vi "Bundle.vi"(8 "error in (no error)":errorcluster, 10 "Actor":refnum<class "Actor.lvclass">, 11 "Launch Subscriber Msg in":refnum<class "Launch Subscriber Msg.lvclass">) -> (0 "error out":errorcluster, 3 "Launch Subscriber Msg out":refnum<class "Launch Subscriber Msg.lvclass">)   [LabVIEW 2020, in "Publisher.lvlib" / "Launch Subscriber Msg.lvclass"]
doc: "Populate the Launc Subscriber Msg class."
uses:
  Launch Subscriber Msg.lvclass
  PPL/HDH.Actor Framework.Core.Actor.lvlibp/1abvi3w/vi.lib/ActorFramework/Actor/Actor.lvclass
  Launch Subscriber Msg.lvclass/Launch Subscriber Msg.ctl
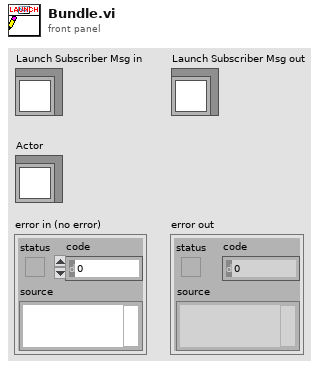
[diagram p1: front panel]
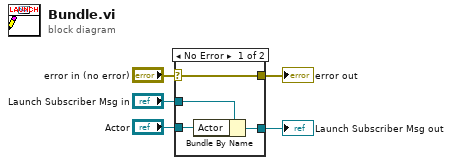
[diagram p0: block diagram]
diagram:
  n1 = case shown="No Error" "error in (no error)" {
    selector: "error in (no error)" -> [w9 w10]
    tunnel: [w9 w10] -> w4
    tunnel: [w7 w11] -> w2
    tunnel: "Launch Subscriber Msg in" -> [w8 w11]
    tunnel: "Actor" -> [w6 _]
    frame No Error {
      n2 = Bundle By Name(cluster=w8, "Actor"=w6) -> (w7:refnum<class "Launch Subscriber Msg.lvclass">)
    }
    frame Error {
    }
  }
  "error out" <- w4
  "Launch Subscriber Msg out" <- w2
